vi "fake Servo modue.vi"(8 "Queue to UI":T5, 11 "Module queue servo":T5) -> ()   [LabVIEW 2024, in "Servo drive module.lvlib"]
doc: "This is TOP VI for Servo control.\n\nCommands:\nInitialize ( ) - Open connections to drivers by ethernet, and gets \nUpdate( ) - Get actual position and makes calculations if something changed\nMove(relative position, axis) - moves by defined step\nEnd( )\n\nResponses: \nStatus changed (quick status[IP addr, Connection, connected, Name, powered, act pos., desir. pos.])\nInitialized (status[connected, powered, act pos., desir. pos.])\nError ... (error cluster) - adds \"error\" before casual response"
uses:
  Servo drive module.lvlib
  Messenger service/Data types/Mailbox address.ctl
  ctl/Servo state.ctl
  ctl/Servo variables.ctl
  ctl/Servo constants.ctl
  ctl/Axis names.ctl
  ctl/Servo MSG.ctl
  ctl/Servo commands.ctl
  Messenger service/Data types/Module name.ctl
  Messenger service/MessengerLib.lvlib
panel:
  in  "Servo statuses":T1[](array[typedef])
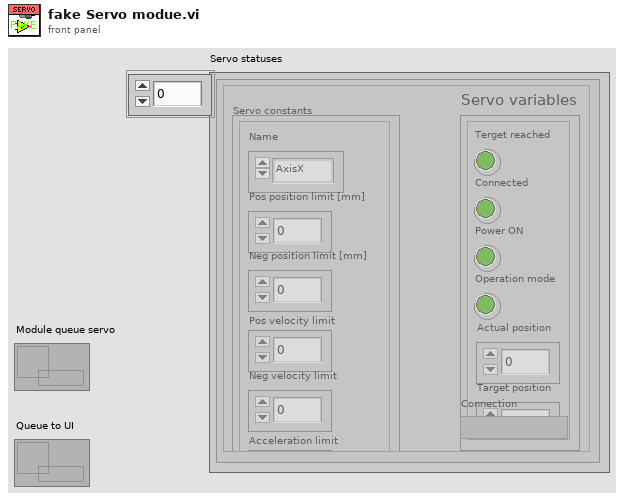
[diagram p1: front panel]
types:
  T1 = typedef "Servo drive module.lvlib/Servo state.ctl" = cluster{"Servo variables":T2, "Servo constants":T3, "Connection":variant}
  T2 = typedef "Servo drive module.lvlib/Servo variables.ctl" = cluster{"Terget reached":bool, "Connected":bool, "Power ON":bool, "Operation mode":bool, "Actual position":dbl, "Target position":dbl}
  T3 = typedef "Servo drive module.lvlib/Servo constants.ctl" = cluster{"Name":T4, "Pos position limit [mm]":dbl, "Neg position limit [mm]":dbl, "Pos velocity limit":dbl, "Neg velocity limit":dbl, "Acceleration limit":dbl}
  T4 = typedef "Servo drive module.lvlib/Axis names.ctl" = enum16{"Unknown", "AxisX", "AxisY", "AxisZ_left", "AxisZ_middle", "AxisZ_right"}
  T5 = typedef "MessengerLib.lvlib/Mailbox address.ctl" = refnum<queue>
  T6 = typedef "Module name.ctl" = enum16{"Emty", "Magnet", "VTI", "Excitation", "Servo", "Acquisition", "Rotator", "Digitizer", "SMU2450", "Carousel", "Multimeter", "Tmp monitor", "Power monitor"}
  T7 = typedef "Servo drive module.lvlib/Servo MSG.ctl" = cluster{"Command":T8, "Data":variant}
  T8 = typedef "Servo drive module.lvlib/Servo commands.ctl" = enum16{"Initialize", "Update", "Move by", "Move to", "Stop", "Ignore", "Disconnect", "End"}
  T9 = typedef "Servo drive module.lvlib/Status variable change.ctl" = cluster{"Property":string, "Value":variant, "Name":T4}
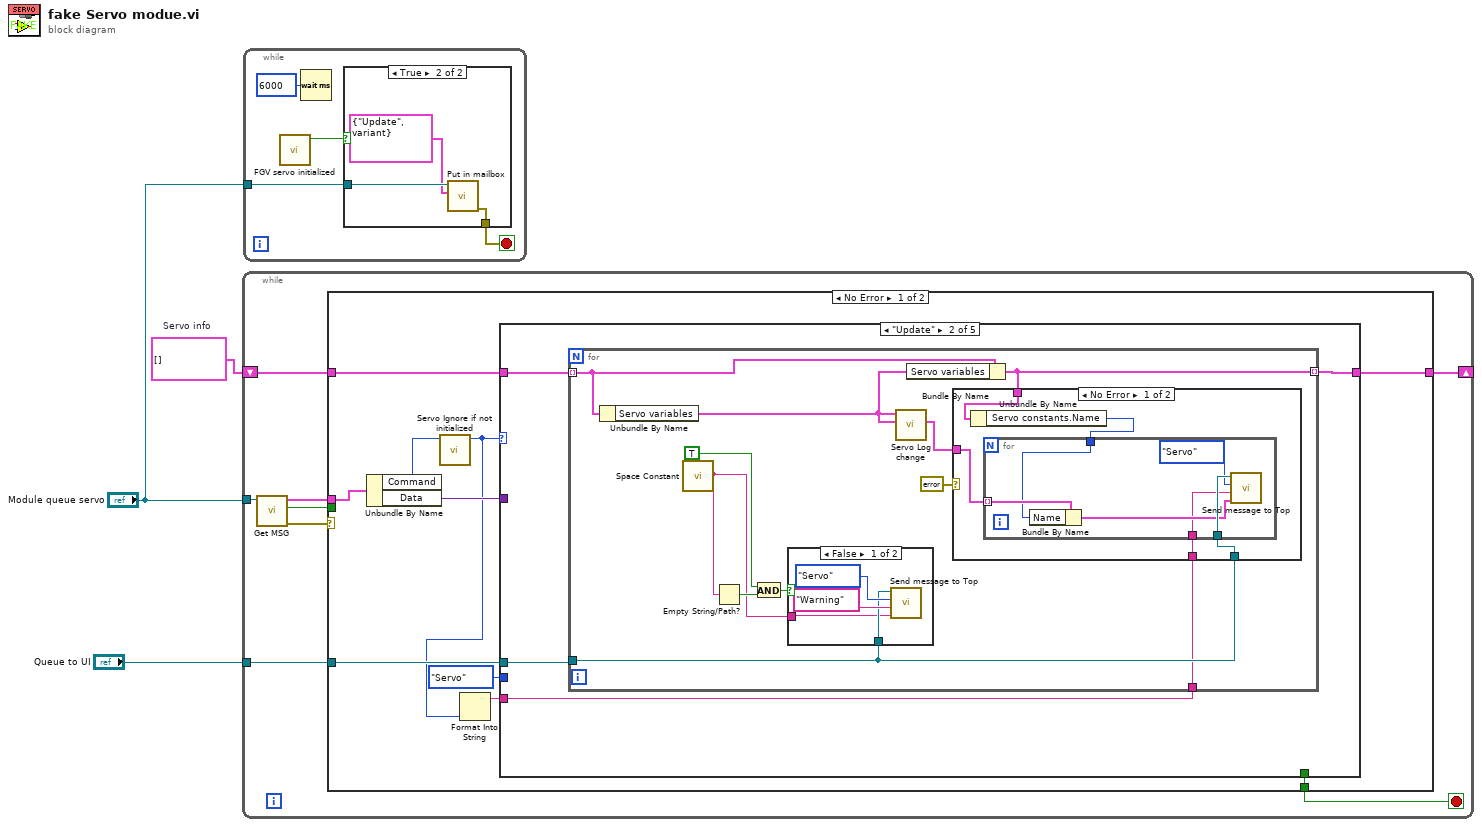
[diagram p0: block diagram]
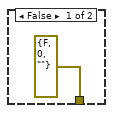
[diagram p2: hidden frame]
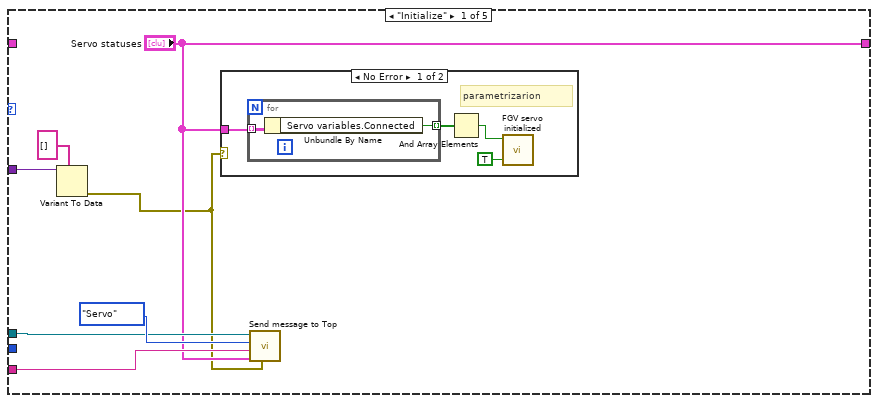
[diagram p3: hidden frame]
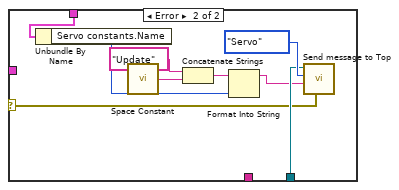
[diagram p6: hidden frame]
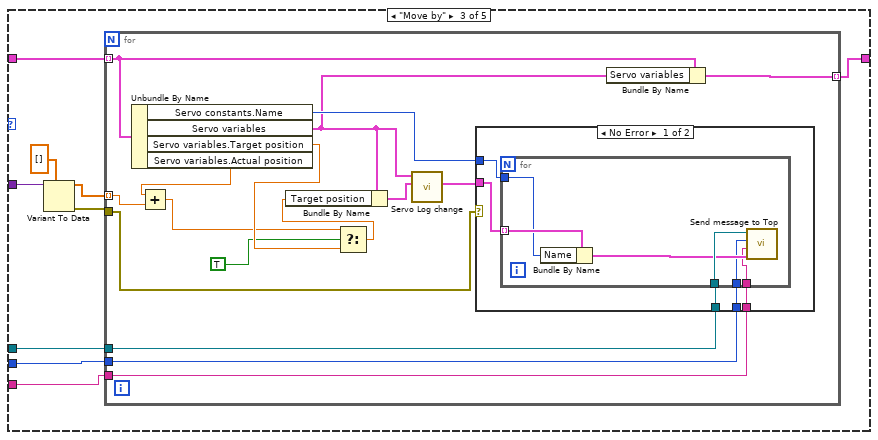
[diagram p7: hidden frame]
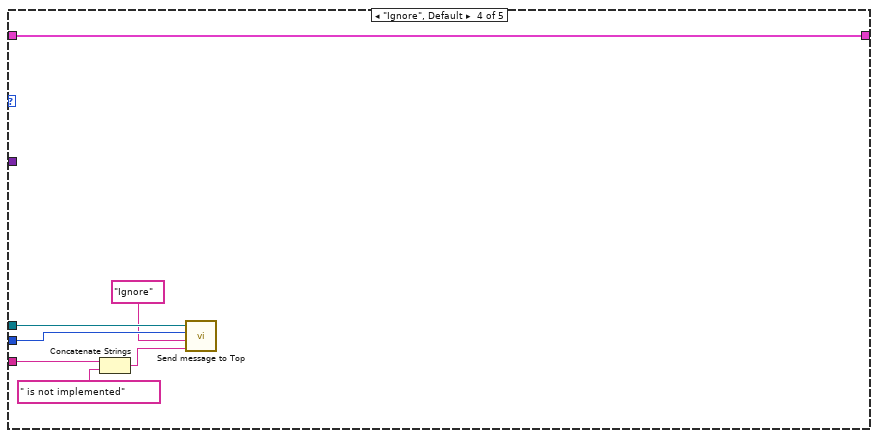
[diagram p9: hidden frame]
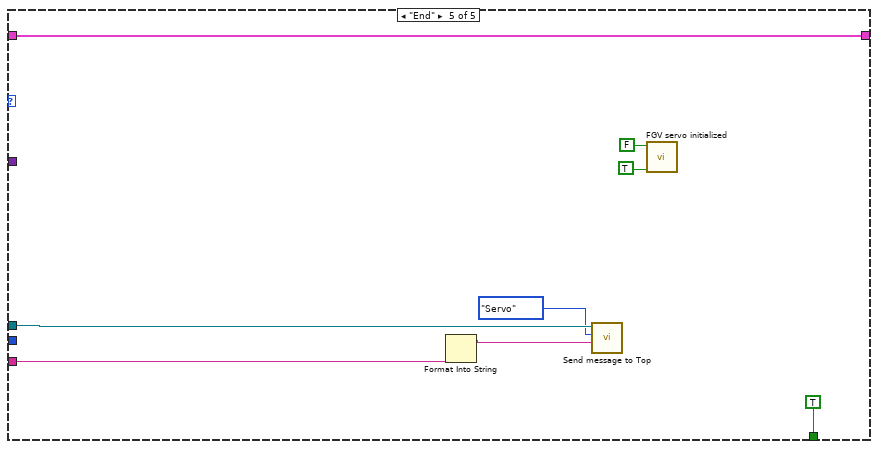
[diagram p10: hidden frame]
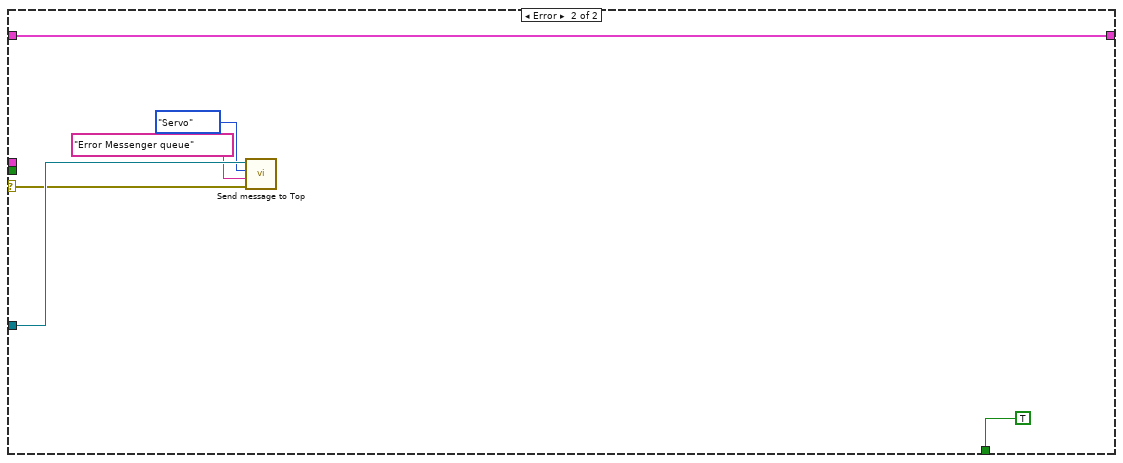
[diagram p11: hidden frame]
diagram:
  w2 = T1[] []  # Servo info
  n1 = while {
    tunnel: "Queue to UI" -> [w11]
    tunnel: "Module queue servo" -> [w10]
    shift-right: [w8] -> _
    shift-left: w2 -> [w9]
    stop <- w5 stop-if-true
    n2 = call "Get MSG.vi"("Queue in"=w10) -> ("error out"=w4:errorcluster, "more than five"=w7:bool, "MSG for servo"=w6:T7)  [unwired: 8 in]
    n3 = case shown="No Error" w4 {
      selector: w4 -> [_ w125]
      tunnel: w7 -> [_ _]
      tunnel: w6 -> [w21 _]
      tunnel: w9 -> [w19 w127]
      tunnel: [w18 w127] -> w8
      tunnel: w11 -> [w17 w130]
      tunnel: [w15 TRUE] -> w5
      frame No Error {
        n4 = Unbundle By Name(w21) -> ("Command"=w16:T8, "Data"=w20:variant)
        n5 = call "Servo Ignore if not initialized.vi"("Command in"=w16) -> ("command out"=w12:T8)  [unwired: 10 in]
        n6 = Format Into String(w12) -> (resulting string=w13:string)  [unwired: 3 in, 1 out]
        n7 = case shown="\"Update\"" w12 {
          tunnel: w20 -> [w26 _ w79 _ _]
          tunnel: w19 -> [_ w38 w81 w116 w121]
          tunnel: ["Servo statuses" w37 w80 w116 w121] -> w18
          tunnel: w17 -> [w27 w36 w82 w115 w120]
          tunnel: [_ _ _ _ TRUE] -> w15
          tunnel: Module_name."Servo" ("Module") -> [_ _ w75 w114 _]
          tunnel: w13 -> [w24 w35 w74 w111 w117]
          frame "Initialize" {
            n8 = Variant To Data(type=string[] [], Variant=w26) -> (error out=w22:errorcluster)  [unwired: 1 in, 1 out]
            n9 = case shown="No Error" w22 {
              tunnel: "Servo statuses" -> [w30 _]
              frame No Error {
                # "parametrizarion"
                n10 = for {
                  tunnel: w30 -> [w34] mode=indexing
                  tunnel: [w33] -> w29 mode=indexing
                  n11 = Unbundle By Name(w34) -> ("Servo variables.Connected"=w33:bool)
                }
                n12 = And Array Elements(Boolean array=w29) -> (logical AND=w31:bool)
                n13 = call "FGV servo initialized.vi"("Write?(F)"=TRUE, "Initialized in"=w31) -> ()  [unwired: 9 in, 1 out]
              }
              frame Error {
              }
            }
            n14 = call "Send message to Top.vi"("Error in (no error)"=w22, "Data"="Servo statuses", "Response"=w24, "Module"=Module_name."Servo", "Mailbox address in"=w27) -> ()  [unwired: 5 in, 2 out]
          }
          frame "Update" {
            n15 = for {
              tunnel: w36 -> [w47]
              tunnel: w38 -> [w46] mode=indexing
              tunnel: [w45] -> w37 mode=indexing
              tunnel: w35 -> [w43]
              n16 = Unbundle By Name(w46) -> ("Servo variables"=w40:T2)
              n17 = call <vilib>:"Space Constant.vi"() -> ("String"=w42:string)
              n18 = Empty String/Path?(string/path=w42) -> (empty?=w48:bool)
              n19 = And(x=TRUE, y=w48) -> (x .and. y?=w49:bool)
              n20 = case shown="False" w49 {
                tunnel: w47 -> [w51 _]
                tunnel: w42 -> [w50 _]
                frame False {
                  n21 = call "Send message to Top.vi"("Data"=w50, "Response"="Warning", "Module"=Module_name."Servo", "Mailbox address in"=w51) -> ()  [unwired: 6 in, 2 out]
                }
                frame True {
                }
              }
              n22 = call "Servo Log change.vi"("Servo variables Now"=w40, "Servo variables Before"=w40) -> ("Changes"=w44:T9[])  [unwired: 8 in, 1 out]
              n23 = Bundle By Name(cluster=w46, "Servo variables"=w40) -> (w45:T1)
              n24 = case shown="No Error" errorcluster {"status"=FALSE, "code"=0, "source"=""} ("error IO") {
                selector: errorcluster {"status"=FALSE, "code"=0, "source"=""} ("error IO") -> [_ w70]
                tunnel: w47 -> [w57 w71]
                tunnel: w45 -> [w56 w69]
                tunnel: w44 -> [w58 _]
                tunnel: w43 -> [w54 _]
                frame No Error {
                  n25 = Unbundle By Name(w56) -> ("Servo constants.Name"=w55:T4)
                  n26 = for {
                    tunnel: w58 -> [w62] mode=indexing
                    tunnel: w57 -> [w64]
                    tunnel: w55 -> [w60]
                    tunnel: w54 -> [w59]
                    n27 = Bundle By Name(cluster=w62, "Name"=w60) -> (w61:T9)
                    n28 = call "Send message to Top.vi"("Data"=w61, "Response"=w59, "Module"=Module_name."Servo", "Mailbox address in"=w64) -> ()  [unwired: 6 in, 2 out]
                  }
                }
                frame Error {
                  n29 = Unbundle By Name(w69) -> ("Servo constants.Name"=w67:T4)
                  n30 = call <vilib>:"Space Constant.vi"() -> ("String"=w73:string)
                  n31 = Concatenate Strings("Update" ("Response"), w73) -> (w66:string)
                  n32 = Format Into String(initial string=w66, w67) -> (resulting string=w65:string)  [unwired: 2 in, 1 out]
                  n33 = call "Send message to Top.vi"("Error in (no error)"=w70, "Response"=w65, "Module"=Module_name."Servo", "Mailbox address in"=w71) -> ()  [unwired: 6 in, 2 out]
                }
              }
            }
          }
          frame "Move by" {
            n34 = Variant To Data(type=dbl[] [], Variant=w79) -> (data=w78:dbl[], error out=w76:errorcluster)  [unwired: 1 in]
            n35 = for {
              tunnel: w82 -> [w98]
              tunnel: w78 -> [w89] mode=indexing
              tunnel: w81 -> [w87] mode=indexing
              tunnel: [w97] -> w80 mode=indexing
              tunnel: w76 -> [w86]
              tunnel: w75 -> [w93]
              tunnel: w74 -> [w92]
              n36 = Unbundle By Name(w87) -> ("Servo constants.Name"=w95:T4, "Servo variables"=w85:T2, "Servo variables.Target position"=w94:dbl, "Servo variables.Actual position"=w88:dbl)
              n37 = Add(x=w88, y=w89) -> (x+y=w90:dbl)
              n38 = Select(t=w90, s=TRUE, f=w94) -> (s? t:f=w84:dbl)
              n39 = Bundle By Name(cluster=w85, "Target position"=w84) -> (w83:T2)
              n40 = call "Servo Log change.vi"("Servo variables Now"=w83, "Servo variables Before"=w85) -> ("Changes"=w96:T9[])  [unwired: 8 in, 1 out]
              n41 = case shown="No Error" w86 {
                tunnel: w98 -> [w103 _]
                tunnel: w96 -> [w102 _]
                tunnel: w95 -> [w101 _]
                tunnel: w93 -> [w100 _]
                tunnel: w92 -> [w99 _]
                frame No Error {
                  n42 = for {
                    tunnel: w103 -> [w109]
                    tunnel: w102 -> [w108] mode=indexing
                    tunnel: w101 -> [w106]
                    tunnel: w100 -> [w105]
                    tunnel: w99 -> [w104]
                    n43 = Bundle By Name(cluster=w108, "Name"=w106) -> (w107:T9)
                    n44 = call "Send message to Top.vi"("Data"=w107, "Response"=w104, "Module"=w105, "Mailbox address in"=w109) -> ()  [unwired: 6 in, 2 out]
                  }
                }
                frame Error {
                }
              }
              n45 = Bundle By Name(cluster=w87, "Servo variables"=w85) -> (w97:T1)
            }
          }
          frame "Ignore", Default {
            n46 = Concatenate Strings(w111, " is not implemented") -> (w112:string)
            n47 = call "Send message to Top.vi"("Data"=w112, "Response"="Ignore", "Module"=w114, "Mailbox address in"=w115) -> ()  [unwired: 6 in, 2 out]
          }
          frame "End" {
            n48 = Format Into String(w117) -> (resulting string=w118:string)  [unwired: 3 in, 1 out]
            n49 = call "Send message to Top.vi"("Response"=w118, "Module"=Module_name."Servo", "Mailbox address in"=w120) -> ()  [unwired: 7 in, 2 out]
            n50 = call "FGV servo initialized.vi"("Write?(F)"=TRUE ("Initialized in"), "Initialized in"=FALSE) -> ()  [unwired: 9 in, 1 out]
          }
        }
      }
      frame Error {
        n51 = call "Send message to Top.vi"("Data"=w125, "Response"="Error Messenger queue", "Module"=Module_name."Servo", "Mailbox address in"=w130) -> ()  [unwired: 6 in, 2 out]
      }
    }
  }
  n52 = while {
    tunnel: "Module queue servo" -> [w132]
    stop <- w131 stop-if-true
    n53 = call "FGV servo initialized.vi"() -> ("Initialized out"=w133:bool)  [unwired: 11 in]
    n54 = Wait (ms)(milliseconds to wait=u32 6000) -> ()  [unwired: 1 out]
    n55 = case shown="True" w133 {
      tunnel: w132 -> [_ w138]
      tunnel: [errorcluster {"status"=FALSE, "code"=0, "source"=""} ("error out") w137] -> w131
      frame False {
      }
      frame True {
        n56 = call "Put in mailbox.vi"("Message"=T7 {"Command"=enum."Update", "Data"=variant(dbl[] [])} ("MSG to Servo"), "Queue in"=w138) -> ("error out"=w137:errorcluster)  [unwired: 7 in, 2 out]
      }
    }
  }
